vi "Initialize.vi"(8 "error in (no error)":errorcluster, 11 "Mettler Settings in":T1) -> (0 "error out":errorcluster, 2 "No Scale Connected":bool, 3 "Mettler Settings out":T1)   [LabVIEW 2018, in "Mettler Toledo.lvlib"]
uses:
  Mettler Toledo.lvlib
  Controls/Settings Cluster.ctl
  <vilib>/Instr/_visa.llb/VISA Configure Serial Port (Instr).vi
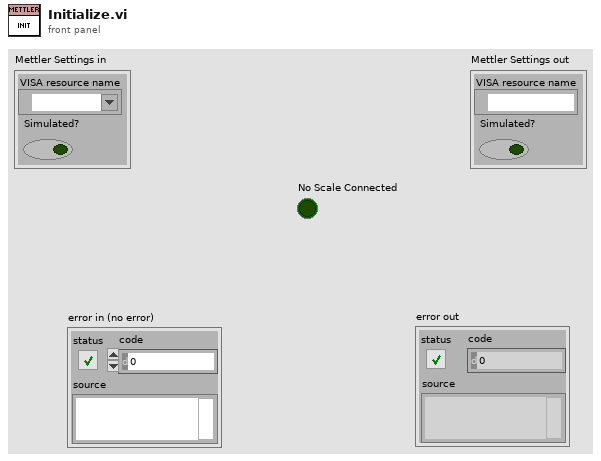
[diagram p1: front panel]
types:
  T1 = typedef "Mettler Toledo.lvlib/Settings Cluster.ctl" = cluster{"VISA resource name":refnum<visa-resource-name>, "Simulated?":bool}
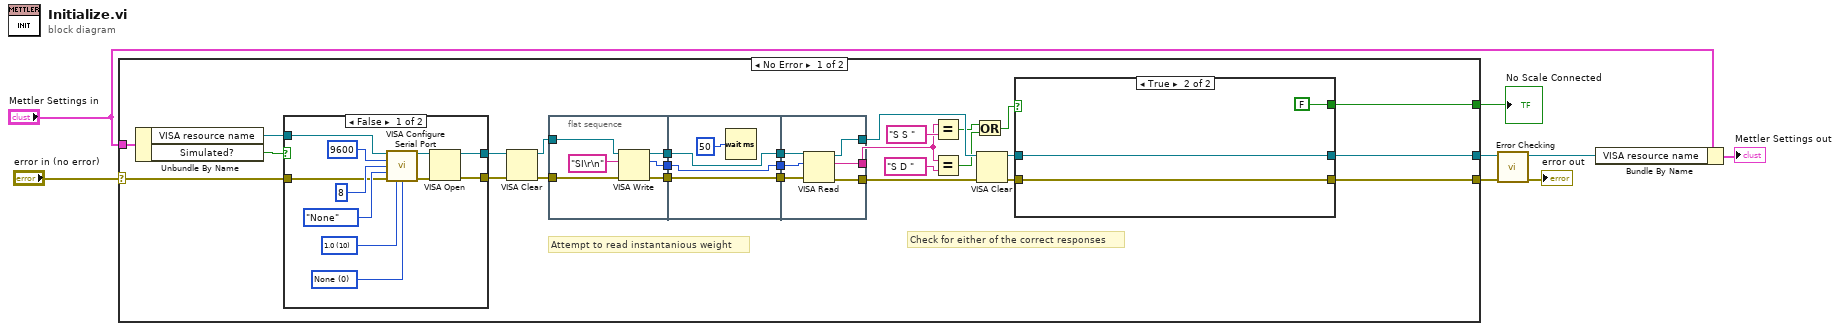
[diagram p0: block diagram]
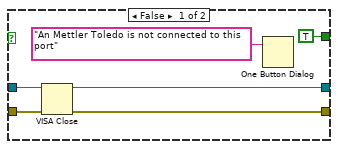
[diagram p2: hidden frame]
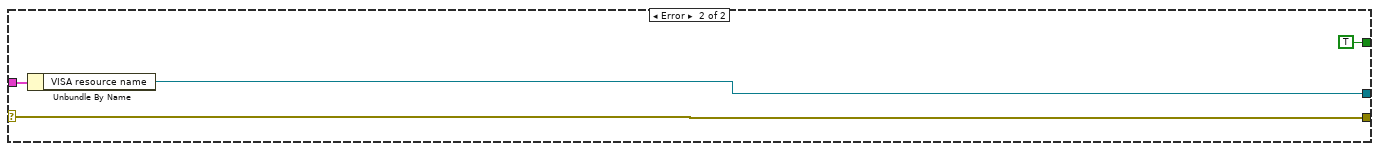
[diagram p4: hidden frame]
diagram:
  n1 = case shown="No Error" "error in (no error)" {
    selector: "error in (no error)" -> [w35 w76]
    tunnel: "Mettler Settings in" -> [w33 w75]
    tunnel: [w29 w76] -> w3
    tunnel: [w30 w74] -> w5
    tunnel: [w9 TRUE] -> w1
    frame No Error {
      # "Check for either of the correct responses"
      # "Attempt to read instantanious weight"
      n2 = Unbundle By Name(w33) -> ("VISA resource name"=w32:refnum<visa-resource-name>, "Simulated?"=w34:bool)
      n3 = case shown="False" w34 {
        tunnel: w35 -> [w64 w72]
        tunnel: [w60 w72] -> w21
        tunnel: [w61 w71] -> w22
        tunnel: w32 -> [w62 w71]
        frame False {
          w66 = u16 0 items=["None", "XON/XOFF", "RTS/CTS", "XON/XOFF & RTS/CTS", "DTR/DSR", "XON/XOFF & DTR/DSR"] ("flow control (0:none)")
          w67 = u16 10 items=["1.0"=10, "1.5"=15, "2.0"=20] ("stop bits (10: 1 bit)")
          n4 = call-poly "VISA Configure Serial Port"("VISA resource name"=w62, "baud rate (9600)"=u32 9600, "data bits (8)"=u16 8, "parity (0:none)"=enum16{"None", "Odd", "Even", "Mark", "Space"}."None", "error in (no error)"=w64, "stop bits (10: 1 bit)"=w67, "flow control (0:none)"=w66) -> ("VISA resource name out"=w63:refnum<visa-resource-name>, "error out"=w65:errorcluster)  [unwired: 7 in]
          n5 = VISA Open(error in (no error)=w65, VISA resource name=w63) -> (VISA resource name=w61:refnum<visa-resource-name>, error out=w60:errorcluster)  [unwired: 3 in]
        }
        frame True {
        }
      }
      n6 = VISA Clear(VISA resource name=w22, error in (no error)=w21) -> (VISA resource name out=w20:refnum<visa-resource-name>, error out=w19:errorcluster)
      n7 = flat-sequence {
        tunnel: w19 -> [w41]
        tunnel: w20 -> [w40]
        tunnel: [w38] -> w28
        tunnel: [w37] -> w26
        tunnel: [w36] -> w17
        tunnel: w28 -> [w45]
        tunnel: [w45] -> w27
        tunnel: w26 -> [w44]
        tunnel: [w44] -> w25
        tunnel: [w42] -> w18
        tunnel: w17 -> [w42]
        tunnel: [w51] -> w15
        tunnel: [w50] -> w13
        tunnel: [w49] -> w16
        tunnel: w27 -> [w48]
        tunnel: w25 -> [w47]
        tunnel: w18 -> [w46]
        frame #0 {
          n8 = VISA Write(VISA resource name=w40, write buffer="SI\r\n", error in (no error)=w41) -> (VISA resource name out=w38:refnum<visa-resource-name>, return count=w36:u32, error out=w37:errorcluster)
        }
        frame #1 {
          n9 = Wait (ms)(milliseconds to wait=u32 50) -> ()  [unwired: 1 out]
        }
        frame #2 {
          n10 = VISA Read(VISA resource name=w48, byte count=w46, error in (no error)=w47) -> (VISA resource name out=w49:refnum<visa-resource-name>, read buffer=w50:string, error out=w51:errorcluster)  [unwired: 1 out]
        }
      }
      n11 = Equal?(x=w13, y="S S ") -> (x = y?=w12:bool)
      n12 = Equal?(x=w13, y="S D ") -> (x = y?=w11:bool)
      n13 = Or(x=w12, y=w11) -> (x .or. y?=w10:bool)
      n14 = VISA Clear(VISA resource name=w16, error in (no error)=w15) -> (VISA resource name out=w24:refnum<visa-resource-name>, error out=w23:errorcluster)
      n15 = case shown="True" w10 {
        tunnel: w24 -> [w54 w59]
        tunnel: w23 -> [w55 w58]
        tunnel: [w54 w59] -> w30
        tunnel: [w53 w58] -> w29
        tunnel: [TRUE FALSE] -> w9
        frame False {
          n16 = VISA Close(VISA resource name=w54, error in (no error)=w55) -> (error out=w53:errorcluster)
          n17 = One Button Dialog(message="An Mettler Toledo is not connected to this port") -> ()  [unwired: 1 in, 1 out]
        }
        frame True {
        }
      }
    }
    frame Error {
      n18 = Unbundle By Name(w75) -> ("VISA resource name"=w74:refnum<visa-resource-name>)
    }
  }
  "No Scale Connected" <- w1
  n19 = call "Error Checking.vi"("error in (no error)"=w3, "VISA resource name"=w5) -> ("error out"=→"error out":errorcluster, "VISA resource name"=w4:refnum<visa-resource-name>)  [unwired: 7 in, 1 out]
  n20 = Bundle By Name(cluster="Mettler Settings in", "VISA resource name"=w4) -> (→"Mettler Settings out":T1)
